vi "SLM Constant.vi"(0 "Ini. Mark In":bool) -> (10 "Monitor Lateral Pixels":i32=1280, 11 "Monitor Count":i32=1280, 12 "Lateral Pixel Number":i32=1280, 13 "Ini. Mark Out":bool, 14 "Lateral Effective Pixel Number":i32=1272, 15 "Vertical (Effective) Pixel Number":i32=1280, 16 "Gray Level Corresponding to 2Pi":i32=1280, 17 "Hologram Coordinate X":i32=1280, 18 "Hologram Coordinate Y":i32=1280, 19 "Hologram Size (px)":i32=1280)   [LabVIEW 2018]
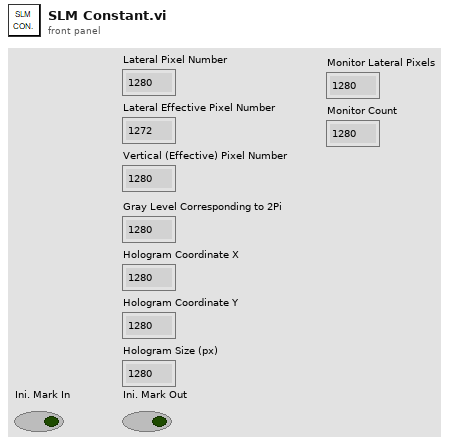
[diagram p1: front panel]
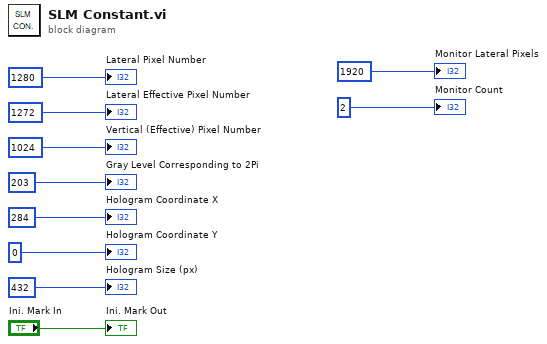
[diagram p0: block diagram]
diagram:
  "Lateral Pixel Number" <- 1280
  "Lateral Effective Pixel Number" <- 1272
  "Vertical (Effective) Pixel Number" <- 1024
  "Gray Level Corresponding to 2Pi" <- 203
  "Hologram Coordinate X" <- 284
  "Hologram Coordinate Y" <- 0
  "Hologram Size (px)" <- 432
  "Ini. Mark Out" <- "Ini. Mark In"
  "Monitor Lateral Pixels" <- 1920
  "Monitor Count" <- 2
